vi "Log Data.vi"(7 "Command":enum16{"Initialize", "Write", "Stop"}(ring), 8 "error in (no error)":errorcluster, 9 "Event Data":string[](array[string]), 11 "file path":path) -> (0 "error out":errorcluster)   [LabVIEW 2013]
uses:
  <vilib>/Utility/file.llb/Write To Spreadsheet File (string).vi
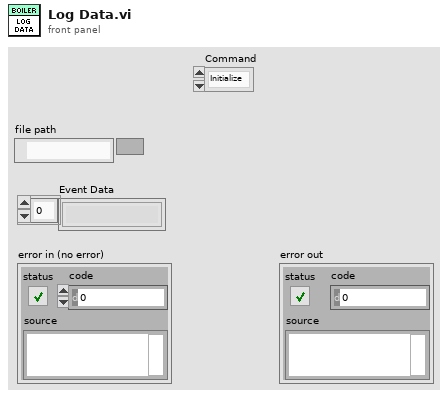
[diagram p1: front panel]
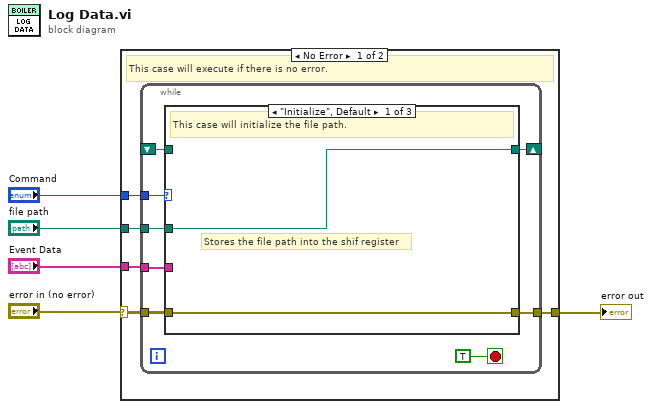
[diagram p0: block diagram]
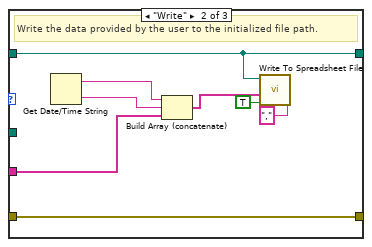
[diagram p2: hidden frame]
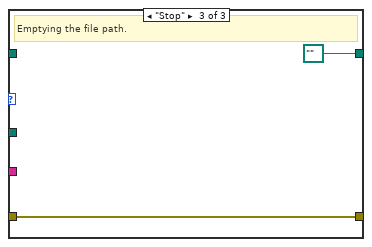
[diagram p3: hidden frame]
diagram:
  n1 = case shown="No Error" "error in (no error)" {
    selector: "error in (no error)" -> [w7 w31]
    tunnel: "Command" -> [w10 _]
    tunnel: "file path" -> [w9 _]
    tunnel: "Event Data" -> [w8 _]
    tunnel: [w6 w31] -> w5
    frame No Error {
      # "This case will execute if there is no error."
      n2 = while {
        tunnel: w10 -> [w17]
        tunnel: w9 -> [w16]
        shift-right: [w15] -> _
        shift-left: _ -> [w14]
        tunnel: w8 -> [w13]
        tunnel: w7 -> [w12]
        tunnel: [w11] -> w6
        stop <- TRUE stop-if-true
        n3 = case shown="\"Initialize\", Default" w17 {
          tunnel: w16 -> [w20 _ _]
          tunnel: [w20 w28 path "" ("file path")] -> w15
          tunnel: w14 -> [_ w28 _]
          tunnel: w13 -> [_ w25 _]
          tunnel: w12 -> [w19 w21 w29]
          tunnel: [w19 w21 w29] -> w11
          frame "Initialize", Default {
            # "Stores the file path into the shif register"
            # "This case will initialize the file path."
          }
          frame "Write" {
            # "Write the data provided by the user to the initialized file path."
            n4 = Get Date/Time String() -> (date string=w27:string, time string=w26:string)  [unwired: 3 in]
            n5 = Build Array (concatenate)(w27, w26, w25) -> (w24:string[])
            n6 = call-poly <vilib>:"Write To Spreadsheet File.vi"("delimiter (\\t)"="," ("delimiter (\\t)"), "append to file? (new file:F)"=TRUE, "1D data"=w24, "file path (dialog if empty)"=w28) -> ()  [unwired: 4 in, 1 out]
          }
          frame "Stop" {
            # "Emptying the file path."
          }
        }
      }
    }
    frame Error {
      # "This case will execute if there is  error."
    }
  }
  "error out" <- w5
